vi "FlushDataReferenceToFile.vi"(8 "error in (no error)":errorcluster, 9 "Qbus":refnum<class "Qbus.lvclass">, 10 "data":variant, 11 "config":T1) -> (0 "error out":errorcluster)   [LabVIEW 2017, in "FileManager.lvlib"]
uses:
  <vilib>/addons/InsightCM/Devices/Shared/Common/FileManager/FileManager.lvlib
  <vilib>/addons/Qbus/Qbus.lvclass
  <vilib>/addons/InsightCM/Devices/Shared/Common/FileManager/controls/config.ctl
  <vilib>/addons/InsightCM/Devices/Shared/Common/DataEvent/DataEvent.lvlib
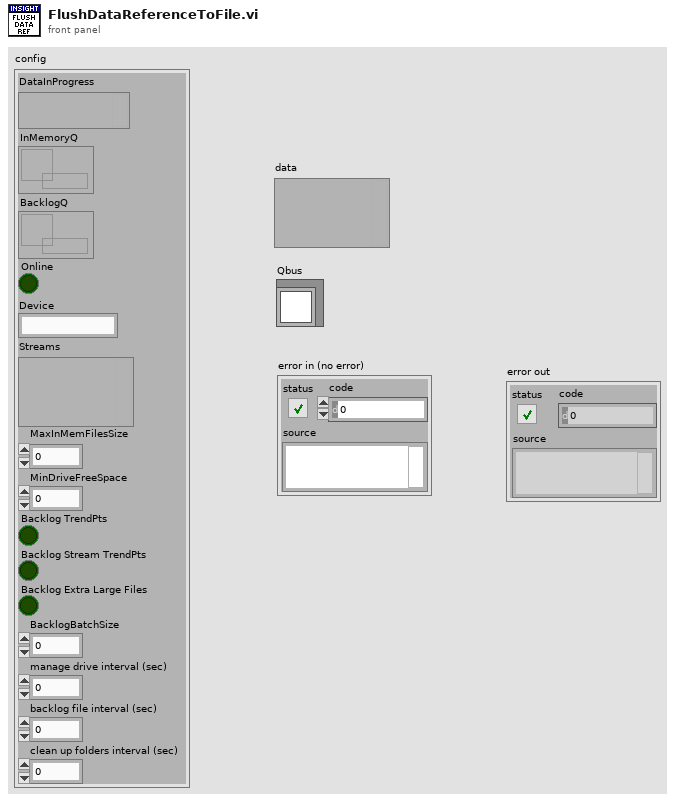
[diagram p1: front panel]
types:
  T1 = typedef "FileManager.lvlib/config.ctl" = cluster{"DataInProgress":variant, "InMemoryQ":refnum<queue>, "BacklogQ":refnum<queue>, "Online":bool, "Device":string, "Streams":variant, "MaxInMemFilesSize":i32, "MinDriveFreeSpace":i32, "Backlog TrendPts":bool, "Backlog Stream TrendPts":bool, "Backlog Extra Large Files":bool, "BacklogBatchSize":i32, "manage drive interval (sec)":dbl, "backlog file interval (sec)":dbl, "clean up folders interval (sec)":dbl}
  T2 = typedef "DataEvent.lvlib/EventReference.ctl" = refnum<data-value>
  T3 = typedef "DataEvent.lvlib/Event.ctl" = cluster{"DataEvent":T4, "DataSets":T6[], "TrendPoints":T8[], "Alarms":T9[]}
  T4 = typedef "DataEvent.ctl" = cluster{"Id":string, "AssetNodeId":string, "Timestamp":i64, "Props":T5[]}
  T5 = typedef "KeyValuePair.ctl" = cluster{"Key":string, "Value":string}
  T6 = typedef "DataEvent.lvlib/DataSet.ctl" = cluster{"DataSetMetadata":T7, "Values":sgl[], "Values DVR":refnum<data-value>}
  T7 = typedef "DataSetMetadata.ctl" = cluster{"Id":string, "DataEventId":string, "AssetNodeId":string, "Type":string, "T0":i64, "Props":T5[]}
  T8 = typedef "TrendPoint.ctl" = cluster{"TrendPointId":string, "DataEventId":string, "Timestamp":i64, "Value":dbl, "Props":T5[]}
  T9 = typedef "TrendAlarmUpdate.ctl" = cluster{"RuleId":string, "Transition":T10}
  T10 = typedef "TrendAlarmTransition.ctl" = cluster{"At":i64, "Severity":i32, "Value":dbl, "Properties":T5[]}
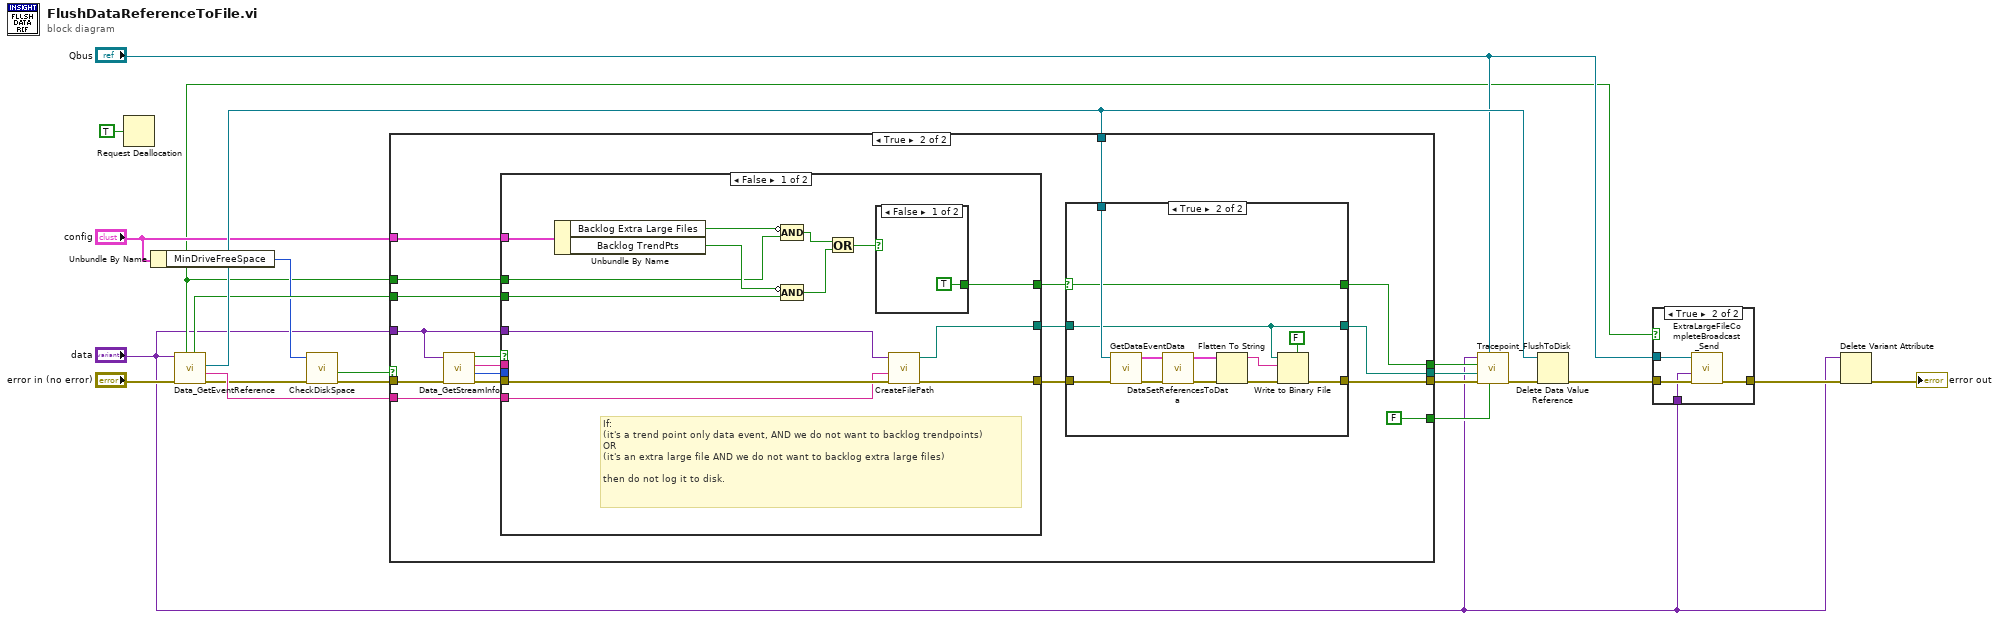
[diagram p0: block diagram]
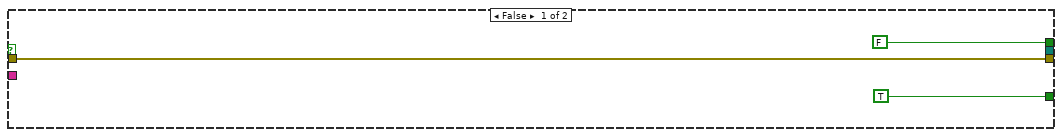
[diagram p3: hidden frame]
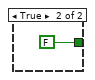
[diagram p5: hidden frame]
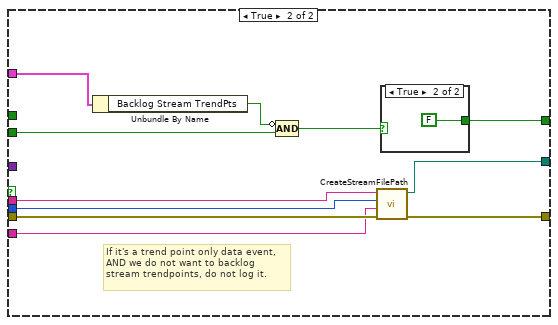
[diagram p6: hidden frame]
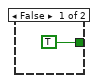
[diagram p7: hidden frame]
diagram:
  n1 = Request Deallocation(TRUE ("flag")) -> ()
  n2 = Unbundle By Name("config") -> ("MinDriveFreeSpace"=w9:i32)
  n3 = call <vilib>:"Data_GetEventReference.vi"("error in (no error)"="error in (no error)", "data"="data") -> ("error out"=w12:errorcluster, "data group"=w20:string, "event reference"=w16:T2, "trend points only"=w15:bool, "extra large file"=w4:bool)  [unwired: 4 in, 1 out]
  n4 = call <vilib>:"CheckDiskSpace.vi"("error in (no error)"=w12, "minimum free disk space"=w9) -> ("error out"=w11:errorcluster, "available disk space"=w8:bool)  [unwired: 6 in, 2 out]
  n5 = case shown="True" w8 {
    tunnel: w20 -> [_ w39]
    tunnel: [w24 w35] -> w19
    tunnel: w16 -> [_ w34]
    tunnel: "data" -> [_ w26]
    tunnel: w15 -> [_ w33]
    tunnel: [_ w31] -> w14
    tunnel: [FALSE w30] -> w13
    tunnel: w11 -> [w24 w29]
    tunnel: "config" -> [_ w28]
    tunnel: [TRUE ("out of disk space") FALSE ("out of disk space")] -> w7
    tunnel: w4 -> [_ w25]
    frame False {
    }
    frame True {
      n6 = call <vilib>:"Data_GetStreamInfo.vi"("error in (no error)"=w29, "data"=w26) -> ("error out"=w41:errorcluster, "block"=w37:i32, "stream Id"=w38:string, "found"=w40:bool)  [unwired: 6 in]
      n7 = case shown="False" w40 {
        tunnel: w41 -> [w69 w84]
        tunnel: [w71 w83] -> w36
        tunnel: [w70 w82] -> w42
        tunnel: w39 -> [w67 w79]
        tunnel: w38 -> [_ w81]
        tunnel: w37 -> [_ w80]
        tunnel: w26 -> [w68 _]
        tunnel: w33 -> [w64 w77]
        tunnel: [w66 w75] -> w32
        tunnel: w28 -> [w63 w78]
        tunnel: w25 -> [w60 _]
        frame False {
          # "If:\n(it's a trend point only data event, AND we do not want to backlog trendpoints)\nOR\n(it's an extra large file AND we do not want to backlog extra large files)\n\nthen do not log it to disk."
          n8 = Unbundle By Name(w63) -> ("Backlog Extra Large Files"=w61:bool, "Backlog TrendPts"=w65:bool)
          n9 = Compound Arithmetic op=AND(invert w61, w60) -> (w59:bool)
          n10 = Compound Arithmetic op=AND(invert w65, w64) -> (w62:bool)
          n11 = Or(x=w59, y=w62) -> (x .or. y?=w58:bool)
          n12 = case shown="False" w58 {
            tunnel: [TRUE FALSE] -> w66
            frame False {
            }
            frame True {
            }
          }
          n13 = call <vilib>:"CreateFilePath.vi"("error in (no error)"=w69, "data group"=w67, "data"=w68) -> ("error out"=w70:errorcluster, "appended path"=w71:path)  [unwired: 7 in]
        }
        frame True {
          # "If it's a trend point only data event,\nAND we do not want to backlog\nstream trendpoints, do not log it."
          n14 = Unbundle By Name(w78) -> ("Backlog Stream TrendPts"=w76:bool)
          n15 = Compound Arithmetic op=AND(invert w76, w77) -> (w74:bool)
          n16 = call <vilib>:"CreateStreamFilePath.vi"("error in (no error)"=w84, "data group"=w79, "block"=w80, "stream id"=w81) -> ("error out"=w82:errorcluster, "file path"=w83:path)  [unwired: 6 in]
          n17 = case shown="True" w74 {
            tunnel: [TRUE FALSE] -> w75
            frame False {
            }
            frame True {
            }
          }
        }
      }
      n18 = case shown="True" w32 {
        selector: w32 -> [w43 w50]
        tunnel: w42 -> [w45 w56]
        tunnel: w36 -> [w44 w51]
        tunnel: [w45 w53] -> w35
        tunnel: w34 -> [_ w52]
        tunnel: [w44 w51] -> w31
        tunnel: [w43 w50] -> w30
        frame False {
        }
        frame True {
          n19 = call <vilib>:"GetDataEventData.vi"("error in (no error)"=w56, "Data Value Reference in"=w52) -> ("error out"=w46:errorcluster, "Data"=w48:T3)  [unwired: 8 in]
          n20 = call <vilib>:"DataSetReferencesToData.vi"("error in (no error)"=w46, "data event"=w48) -> ("error out"=w47:errorcluster, "data event out"=w49:T3)  [unwired: 8 in]
          n21 = Flatten To String(anything=w49, error in (no error)=w47) -> (data string=w54:string, error out=w55:errorcluster)  [unwired: 2 in, 1 out]
          n22 = Write to Binary File(file (use dialog)=w51, data=w54, error in=w55, 5:FALSE ("prepend array or string size? (T)")) -> (error out=w53:errorcluster)  [unwired: 2 in, 2 out]
        }
      }
    }
  }
  n23 = call <vilib>:"Tracepoint_FlushToDisk.vi"("out of disk space"=w7, "Qbus"="Qbus", "error in (no error)"=w19, "file path"=w14, "wrote to disk"=w13, "data"="data") -> ("error out"=w18:errorcluster)  [unwired: 5 in]
  n24 = Delete Data Value Reference(data value reference=w16, error in=w18) -> (error out=w3:errorcluster)  [unwired: 1 out]
  n25 = case shown="True" w4 {
    tunnel: "Qbus" -> [_ w89]
    tunnel: w3 -> [w87 w91]
    tunnel: [w87 w90] -> w2
    tunnel: "data" -> [_ w88]
    frame False {
    }
    frame True {
      n26 = call <vilib>:"ExtraLargeFileCompleteBroadcast_Send.vi"("error in (no error)"=w91, "data"=w88, "Qbus in"=w89) -> ("error out"=w90:errorcluster)  [unwired: 8 in]
    }
  }
  n27 = Delete Variant Attribute(4:w2, 7:"data") -> (0:→"error out":errorcluster)  [unwired: 1 in, 2 out]
